vi "Upper Triangular Matrix (DBL).vi"(10 "k":i32, 11 "A":T1) -> (3 "U":T1)   [LabVIEW 2017, in "NI_AAL_LinAlg.lvlib"]
uses:
  <vilib>/Analysis/NI_AAL_LinAlg.lvlib
  <vilib>/Analysis/Matrix/Datatypes/RealMatrix.ctl
  <vilib>/Analysis/Matrix/NI_Matrix.lvlib
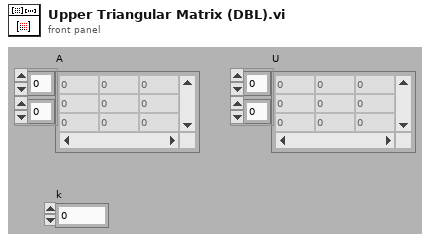
[diagram p1: front panel]
types:
  T1 = typedef "NI_Matrix.lvlib/RealMatrix.ctl" = dbl[][]
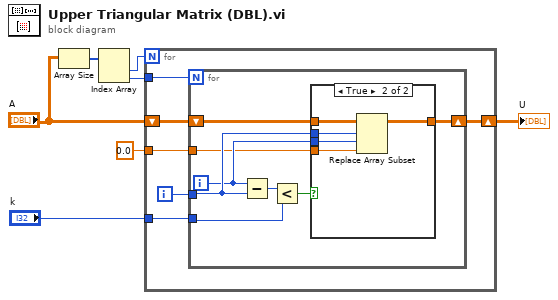
[diagram p0: block diagram]
diagram:
  n1 = Array Size(array="A") -> (size(s)=w6:i32[])
  n2 = Index Array(array=w6) -> (element #1=w5:i32, element #2=w4:i32)  [unwired: 2 in]
  n3 = for {
    N: w5 -> [_]
    shift-right: [w9] -> w3
    shift-left: "A" -> [w13]
    tunnel: w4 -> [w12]
    tunnel: "k" -> [w11]
    tunnel: 0.0 ("DNL_NI_Generic") -> [w8]
    i -> [w10]
    n4 = for {
      N: w12 -> [_]
      shift-right: [w15] -> w9
      shift-left: w13 -> [w16]
      tunnel: w11 -> [w20]
      tunnel: w10 -> [w18]
      tunnel: w8 -> [w14]
      i -> [w17]
      n5 = Subtract(x=w17, y=w18) -> (x-y=w21:i32)
      n6 = Less?(x=w21, y=w20) -> (x < y?=w19:bool)
      n7 = case shown="True" w19 {
        tunnel: w18 -> [_ w26]
        tunnel: w17 -> [_ w25]
        tunnel: w16 -> [w22 w27]
        tunnel: [w22 w24] -> w15
        tunnel: w14 -> [_ w23]
        frame False {
        }
        frame True {
          n8 = Replace Array Subset(array=w27, new element=w23, index (row)=w26, index (col)=w25) -> (w24:T1)
        }
      }
    }
  }
  "U" <- w3
